vi "rvc Set Blend Time.vi"(9 "time steps":dbl, 10 "seg":i32, 11 "acceleration limits":dbl[](array[numeric])) -> (1 "tacc2":dbl, 2 "tacc":dbl, 3 "taccx":dbl)   [LabVIEW 2013]
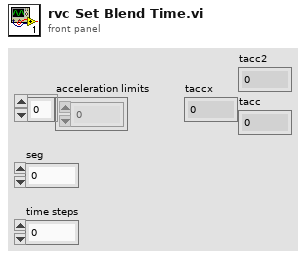
[diagram p1: front panel]
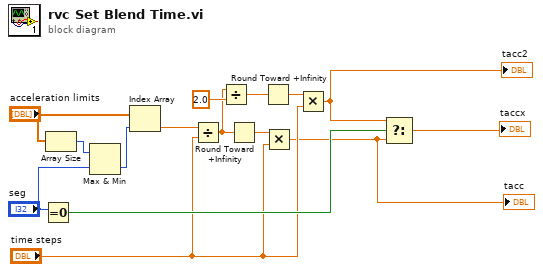
[diagram p0: block diagram]
diagram:
  n1 = Equal To 0?(x="seg") -> (x = 0?=w14:bool)
  n2 = Array Size(array="acceleration limits") -> (size(s)=w2:i32)
  n3 = Max & Min(x=w2, y="seg") -> (min(x,y)=w3:i32)  [unwired: 1 out]
  n4 = Index Array(array="acceleration limits", index=w3) -> (element=w5:dbl)
  n5 = Divide(x=w5, y="time steps") -> (x/y=w9:dbl)
  n6 = Divide(x=w9, y=2.0) -> (x/y=w12:dbl)
  n7 = Round Toward +Infinity(x=w9) -> (ceil(x): smallest int >= x=w8:dbl)
  n8 = Round Toward +Infinity(x=w12) -> (ceil(x): smallest int >= x=w11:dbl)
  n9 = Multiply(x=w8, y="time steps") -> (x*y=w1:dbl)
  "tacc" <- w1
  n10 = Multiply(x=w11, y="time steps") -> (x*y=w13:dbl)
  "tacc2" <- w13
  n11 = Select(t=w13, s=w14, f=w1) -> (s? t:f=→"taccx":dbl)
